vi "TaskMon_CPUload.vi"(7 "SynchronizationRefs":T2, 8 "error in (no error)":errorcluster, 11 "VI Server Cluster":T1={"Refs"=[], "Labels"=["Label", "Size", "Font", "Heght", "Width", "Ledding Denominator", "Ledding Nominator", "Label Number", "Microstep Resolution", "X", "Y", "Z", "Italic?", "Underlined?"], "VI Ref"=refnum}) -> (0 "error out":errorcluster, 4 "return":i32)   [LabVIEW 2020]
uses:
  processHandles.dll
  toolkits_lv2013_32bit/VI Server ToolKit/VIS_Libraries/VI Server_Get Controls.llb/Recover Text Ring DBL.vi
  Synchronization.llb/TaskMon_SynchronizationRef.ctl
  toolkits_lv2013_32bit/VI Server ToolKit/Labels&Control References.ctl
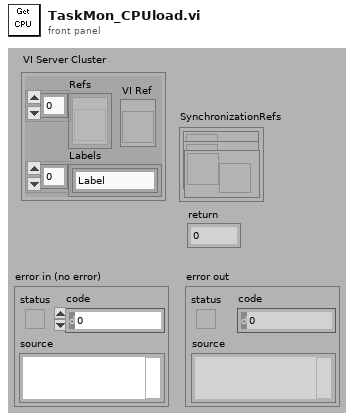
[diagram p1: front panel]
types:
  T1 = typedef "Labels&Control References.ctl" = cluster{"Refs":refnum<vi>[], "Labels":string[], "VI Ref":refnum<vi>}
  T2 = typedef "TaskMon_SynchronizationRef.ctl" = cluster{"STOP":refnum<notifier>, "PID":refnum<notifier>, "Process":refnum<notifier>}
  T3 = cluster{"dwLowDateTime":u32, "dwHighDateTime":u32}
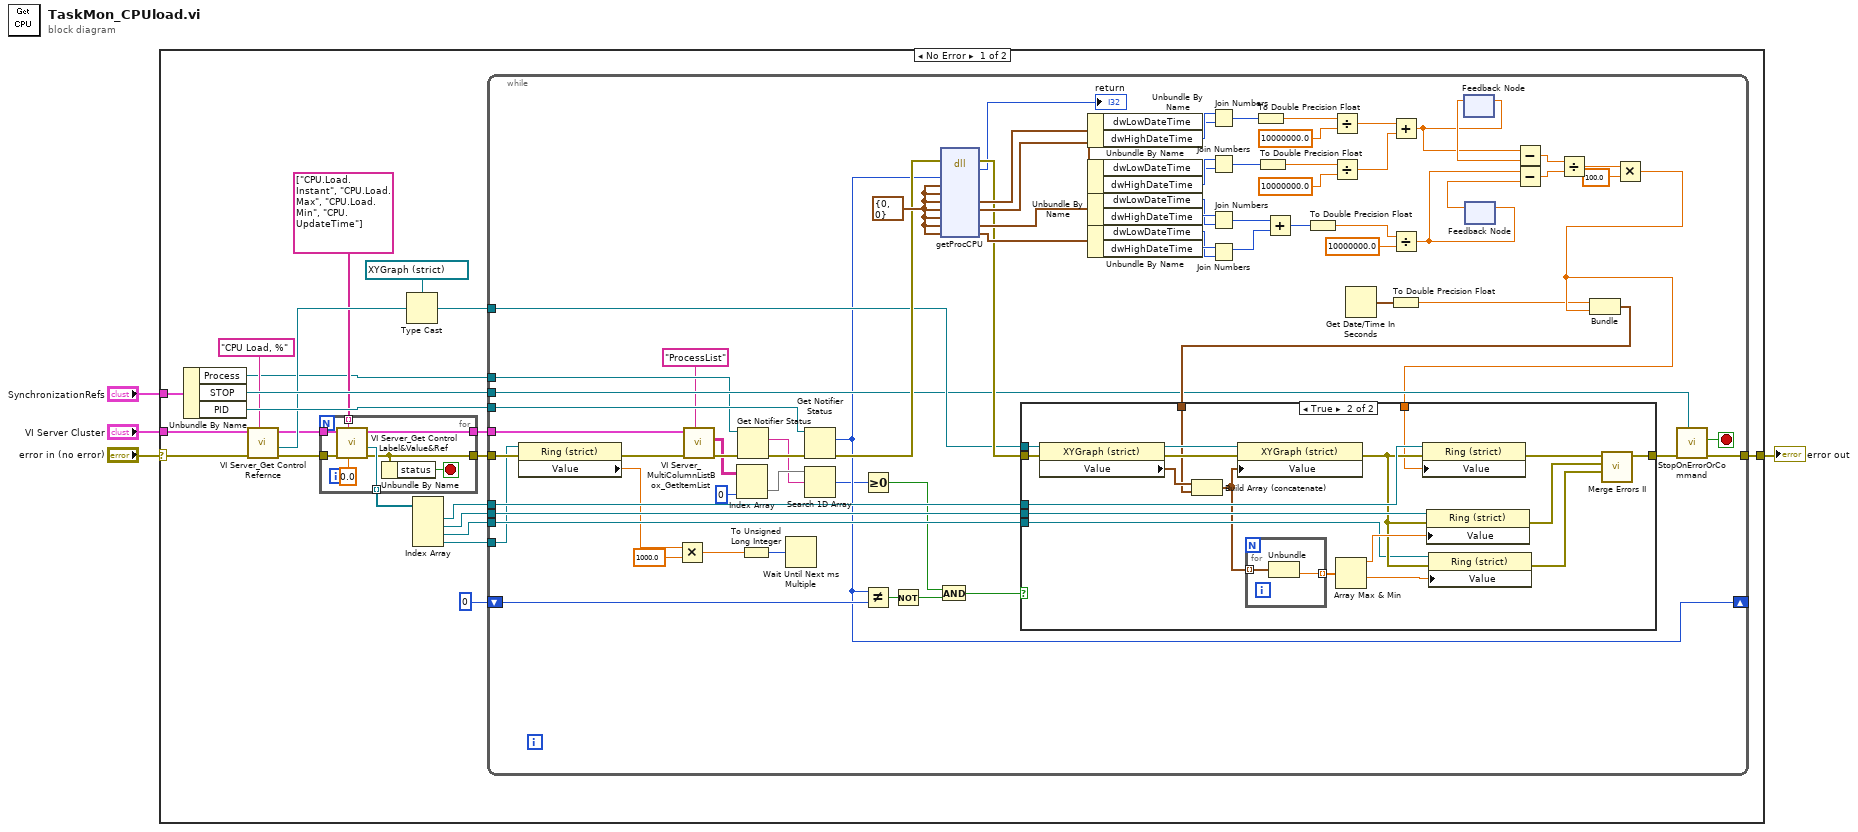
[diagram p0: block diagram]
diagram:
  n1 = case shown="No Error" "error in (no error)" {
    selector: "error in (no error)" -> [w17 w130]
    tunnel: "SynchronizationRefs" -> [w26 _]
    tunnel: "VI Server Cluster" -> [w23 _]
    tunnel: [w18 w130] -> w2
    frame No Error {
      n2 = Unbundle By Name(w26) -> ("Process"=w7:refnum<notifier>, "STOP"=w24:refnum<notifier>, "PID"=w25:refnum<notifier>)
      n3 = call "VI Server_Get Control Refernce.vi"("Label"="CPU Load, %", "error in"=w17, "VI Server Cluster"=w23) -> ("error out"=w16:errorcluster, "Control Reference"=w21:refnum<vi>, "VI Server Cluster DUP"=w14:T1)  [unwired: 5 in, 1 out]
      n4 = for {
        tunnel: w16 -> [w34]
        tunnel: [w30] -> w15
        tunnel: w14 -> [w33]
        tunnel: [w31] -> w11 mode=indexing
        tunnel: string[] ["CPU.Load.Instant", "CPU.Load.Max", "CPU.Load.Min", "CPU.UpdateTime"] -> [w28] mode=indexing
        tunnel: [w27] -> w6
        stop <- w29 stop-if-true
        n5 = call-poly "VI Server_Get Control Label&Value&Ref.vi"("Default Value"=0.0 ("CPU.Load.Instant"), "Label"=w28, "error in"=w34, "Data Cluster"=w33) -> ("error out"=w30:errorcluster, "Control Ref"=w31:refnum<vi>, "Data Cluster dup"=w27:T1)  [unwired: 3 in, 2 out]
        n6 = Unbundle By Name(w30) -> ("status"=w29:bool)
      }
      n7 = Type Cast(type=refnum<vi> refnum ("CPU Load, %"), x=w21) -> (*(type *) &x=w19:refnum<vi>)
      n8 = Index Array(array=w11) -> (element #1=w12:refnum<vi>, element #2=w10:refnum<vi>, element #3=w9:refnum<vi>, element #4=w5:refnum<vi>)  [unwired: 4 in]
      n9 = while {
        tunnel: w25 -> [w77]
        tunnel: w15 -> [w40]
        tunnel: w24 -> [w64]
        tunnel: w19 -> [w69]
        tunnel: [w62] -> w18
        tunnel: w12 -> [w63]
        tunnel: w10 -> [w61]
        tunnel: w9 -> [w60]
        shift-right: [w56] -> _
        shift-left: 0 ("latest notification") -> [w58]
        tunnel: w7 -> [w54]
        tunnel: w6 -> [w52]
        tunnel: w5 -> [w38]
        stop <- w66 stop-if-true
        w73 = T3 {"dwLowDateTime"=0, "dwHighDateTime"=0} ("Cluster")
        n10 = property class="Ring (strict)"(reference=w38, error in=w40) -> (error out=w41:errorcluster, "Value"=w36:dbl)  [unwired: 1 out]
        n11 = Multiply(x=w36, y=1000.0) -> (x*y=w37:dbl)
        n12 = call "VI Server_MultiColumnListBox_GetItemList.vi"("Label"="ProcessList", "error in"=w41, "Data Cluster"=w52) -> ("error out"=w53:errorcluster, "ItemNames"=w48:string[][])  [unwired: 3 in, 4 out]
        n13 = Index Array(array=w48, index (col)=0 ("disabled index (col)")) -> (element=w46:string[])  [unwired: 1 in]
        n14 = Get Notifier Status(notifier=w54, error in (no error)=w53) -> (current notification=w45:string, error out=w55:errorcluster)  [unwired: 3 out]
        n15 = To Unsigned Long Integer(number=w37) -> (unsigned 32bit integer=w39:u32)
        n16 = Wait Until Next ms Multiple(millisecond multiple=w39) -> ()  [unwired: 1 out]
        n17 = Get Notifier Status(notifier=w77, error in (no error)=w55) -> (current notification=w56:i32, error out=w72:errorcluster)  [unwired: 3 out]
        n18 = Search 1D Array(1D array=w46, element=w45) -> (index of element=w44:i32)  [unwired: 1 in]
        n19 = Greater Or Equal To 0?(x=w44) -> (x >= 0?=w43:bool)
        n20 = Not Equal?(x=w56, y=w58) -> (x != y?=w57:bool)
        n21 = Not(x=w57) -> (.not. x?=w50:bool)
        n22 = And(x=w43, y=w50) -> (x .and. y?=w49:bool)
        n23 = dll-call lib="E:/LabVIEW 2020 Toolkits/toolkits_lv2020_32bit/TaskManager/processHandles.dll" fn="getProcCPU"(error in=w72, "arg5"=w56, "arg1"=w73, "arg2"=w73, "arg3"=w73, "arg4"=w73, "arg6"=w73, "arg7"=w73, "arg8"=w73) -> (error out=w70:errorcluster, "return type"=→"return":i32, "arg3"=w107:T3, "arg4"=w104:T3, "arg7"=w93:T3, "arg8"=w92:T3)  [unwired: 3 in, 4 out]
        n24 = Unbundle By Name(w107) -> ("dwLowDateTime"=w105:u32, "dwHighDateTime"=w106:u32)
        n25 = Unbundle By Name(w104) -> ("dwLowDateTime"=w102:u32, "dwHighDateTime"=w103:u32)
        n26 = Unbundle By Name(w93) -> ("dwLowDateTime"=w95:u32, "dwHighDateTime"=w97:u32)
        n27 = Unbundle By Name(w92) -> ("dwLowDateTime"=w94:u32, "dwHighDateTime"=w96:u32)
        n28 = Join Numbers(hi=w106, lo=w105) -> ((hi.lo)=w89:u64)
        n29 = Join Numbers(hi=w103, lo=w102) -> ((hi.lo)=w88:u64)
        n30 = Join Numbers(hi=w97, lo=w95) -> ((hi.lo)=w90:u64)
        n31 = Join Numbers(hi=w96, lo=w94) -> ((hi.lo)=w91:u64)
        n32 = To Double Precision Float(number=w89) -> (double precision float=w76:dbl)
        n33 = To Double Precision Float(number=w88) -> (double precision float=w75:dbl)
        n34 = Add(x=w90, y=w91) -> (x+y=w87:u64)
        n35 = To Double Precision Float(number=w87) -> (double precision float=w74:dbl)
        n36 = Divide(x=w76, y=10000000.0) -> (x/y=w99:dbl)
        n37 = Divide(x=w75, y=10000000.0) -> (x/y=w98:dbl)
        n38 = Get Date/Time In Seconds() -> (seconds since 1Jan1904=w71:timestamp)
        n39 = Add(x=w99, y=w98) -> (x+y=w79:dbl)
        n40 = Divide(x=w74, y=10000000.0) -> (x/y=w78:dbl)
        n41 = To Double Precision Float(number=w71) -> (double precision float=w42:dbl)
        n42 = feedback-in #1(w79) -> ()
        n43 = feedback #1() -> (w85:dbl)  [unwired: 1 in]
        n44 = feedback-in #2(w78) -> ()
        n45 = feedback #2() -> (w80:dbl)  [unwired: 1 in]
        n46 = Subtract(x=w79, y=w85) -> (x-y=w84:dbl)
        n47 = Subtract(x=w78, y=w80) -> (x-y=w81:dbl)
        n48 = Divide(x=w84, y=w81) -> (x/y=w83:dbl)
        n49 = Multiply(x=w83, y=100.0) -> (x*y=w59:dbl)
        n50 = Bundle(w42, w59) -> (w68:cluster{dbl, dbl})  [unwired: 1 in]
        n51 = case shown="True" w49 {
          tunnel: w70 -> [w108 w127]
          tunnel: w69 -> [_ w126]
          tunnel: w68 -> [_ w122]
          tunnel: [w108 w121] -> w67
          tunnel: w63 -> [_ w120]
          tunnel: w61 -> [_ w118]
          tunnel: w60 -> [_ w114]
          tunnel: w59 -> [_ w110]
          frame False {
          }
          frame True {
            n52 = property class="XYGraph (strict)"(reference=w126, error in=w127) -> (reference out=w124:refnum<vi>, error out=w125:errorcluster, "Value"=w123:cluster{dbl, dbl}[])
            n53 = Build Array (concatenate)(w123, w122) -> (w109:cluster{dbl, dbl}[])
            n54 = property class="XYGraph (strict)"(reference=w124, error in=w125, "Value"=w109) -> (error out=w116:errorcluster)  [unwired: 1 out]
            n55 = for {
              tunnel: w109 -> [w129] mode=indexing
              tunnel: [w128] -> w119 mode=indexing
              n56 = Unbundle(w129) -> (w128:dbl)  [unwired: 1 out]
            }
            n57 = Array Max & Min(array=w119) -> (max value=w117:dbl, min value=w115:dbl)  [unwired: 2 out]
            n58 = property class="Ring (strict)"(reference=w120, error in=w116, "Value"=w110) -> (error out=w113:errorcluster)  [unwired: 1 out]
            n59 = property class="Ring (strict)"(reference=w118, error in=w116, "Value"=w117) -> (error out=w112:errorcluster)  [unwired: 1 out]
            n60 = property class="Ring (strict)"(reference=w114, error in=w116, "Value"=w115) -> (error out=w111:errorcluster)  [unwired: 1 out]
            n61 = call "Merge Errors II.vi"("error in 3 (no error)"=w111, "error in 2 (no error)"=w112, "error in 1 (no error)"=w113) -> ("error out.DUP"=w121:errorcluster)  [unwired: 3 in, 1 out]
          }
        }
        n62 = call "StopOnErrorOrCommand.vi"("STOP"=w64, "error in (no error)"=w67) -> ("error out"=w62:errorcluster, "STOP"=w66:bool)  [unwired: 8 in]
      }
    }
    frame Error {
    }
  }
  "error out" <- w2
